vi "HMI.vi"(5 "Disabled?":bool=TRUE, 7 "HMI to Control":T1={"RightDriveValue"=0.0, "LeftDriveValue"=0.0, "Arm Manual "=0.0, "Stacker Manual "=0.0, "Claw Manual "=0.0, "ClawSlightOpenNumber"=0, "Intake Value "=0.0, "Arm States"=enum."4 Tote", "Claw States"=enum."Claw Manual ", "Intake Man. or Sense"=enum."Sensing", "Stacker in Manual?"=FALSE, "Drop Stack? "=FALSE, "Tusk Up Request"=FALSE, "Tusk Down Request"=FALSE, "Inver. Wheels  In Request"=FALSE, "Inverse. Wheels Out Request "=FALSE, "Get Out of Manual Control"=FALSE, "Exit Score State"=FALSE, "DriveStraight Help?"=FALSE, "Stacker Shut Off No."=0, "Stacker Need Off?"=FALSE, "Collecting?"=FALSE, "Go to Hover"=FALSE, "Stack Clamp Lock "=FALSE, "Stack Clamp Unlock "=FALSE, "Claw Intake Value "=0.0, "Stack Clamp Lock No. "=0, "Steal Can (ruin their day?)"=FALSE, "Retract (have mercy?)"=FALSE, "Can Grab No. "=0, "Wench Value to Control "=0.0}, 9 "GamepadData":T5) -> (1 "HMI to Control Out":T1={"RightDriveValue"=0.0, "LeftDriveValue"=0.0, "Arm Manual "=0.0, "Stacker Manual "=0.0, "Claw Manual "=0.0, "ClawSlightOpenNumber"=0, "Intake Value "=0.0, "Arm States"=enum."4 Tote", "Claw States"=enum."Claw Manual ", "Intake Man. or Sense"=enum."Sensing", "Stacker in Manual?"=FALSE, "Drop Stack? "=FALSE, "Tusk Up Request"=FALSE, "Tusk Down Request"=FALSE, "Inver. Wheels  In Request"=FALSE, "Inverse. Wheels Out Request "=FALSE, "Get Out of Manual Control"=FALSE, "Exit Score State"=FALSE, "DriveStraight Help?"=FALSE, "Stacker Shut Off No."=0, "Stacker Need Off?"=FALSE, "Collecting?"=FALSE, "Go to Hover"=FALSE, "Stack Clamp Lock "=FALSE, "Stack Clamp Unlock "=FALSE, "Claw Intake Value "=0.0, "Stack Clamp Lock No. "=0, "Steal Can (ruin their day?)"=FALSE, "Retract (have mercy?)"=FALSE, "Can Grab No. "=0, "Wench Value to Control "=0.0}, 3 "GamepadDataOut":T5)   [LabVIEW 2015]
uses:
  Typedefs/GamepadData.ctl
  Typedefs/HMI_to_Control.ctl
  Typedefs/Arm States.ctl
  Typedefs/ClawStates.ctl
  Typedefs/IntakeWheelSenseOrManual.ctl
  Auton/scriptlib/auto_data.vi
panel:
  in  "Wheel Ramp Step":dbl=1.0 format="%#_13g"
  in  "Throttle Ramp Step":dbl=0.015
  in  "Claw Man Threshold":dbl=0.2
  in  "Throttle Drive Straight Assist Threshold":dbl=0.2
  in  "Wheel Drive Straight Assist Threshold":dbl=0.15
  in  "Man Threshold":dbl=0.3
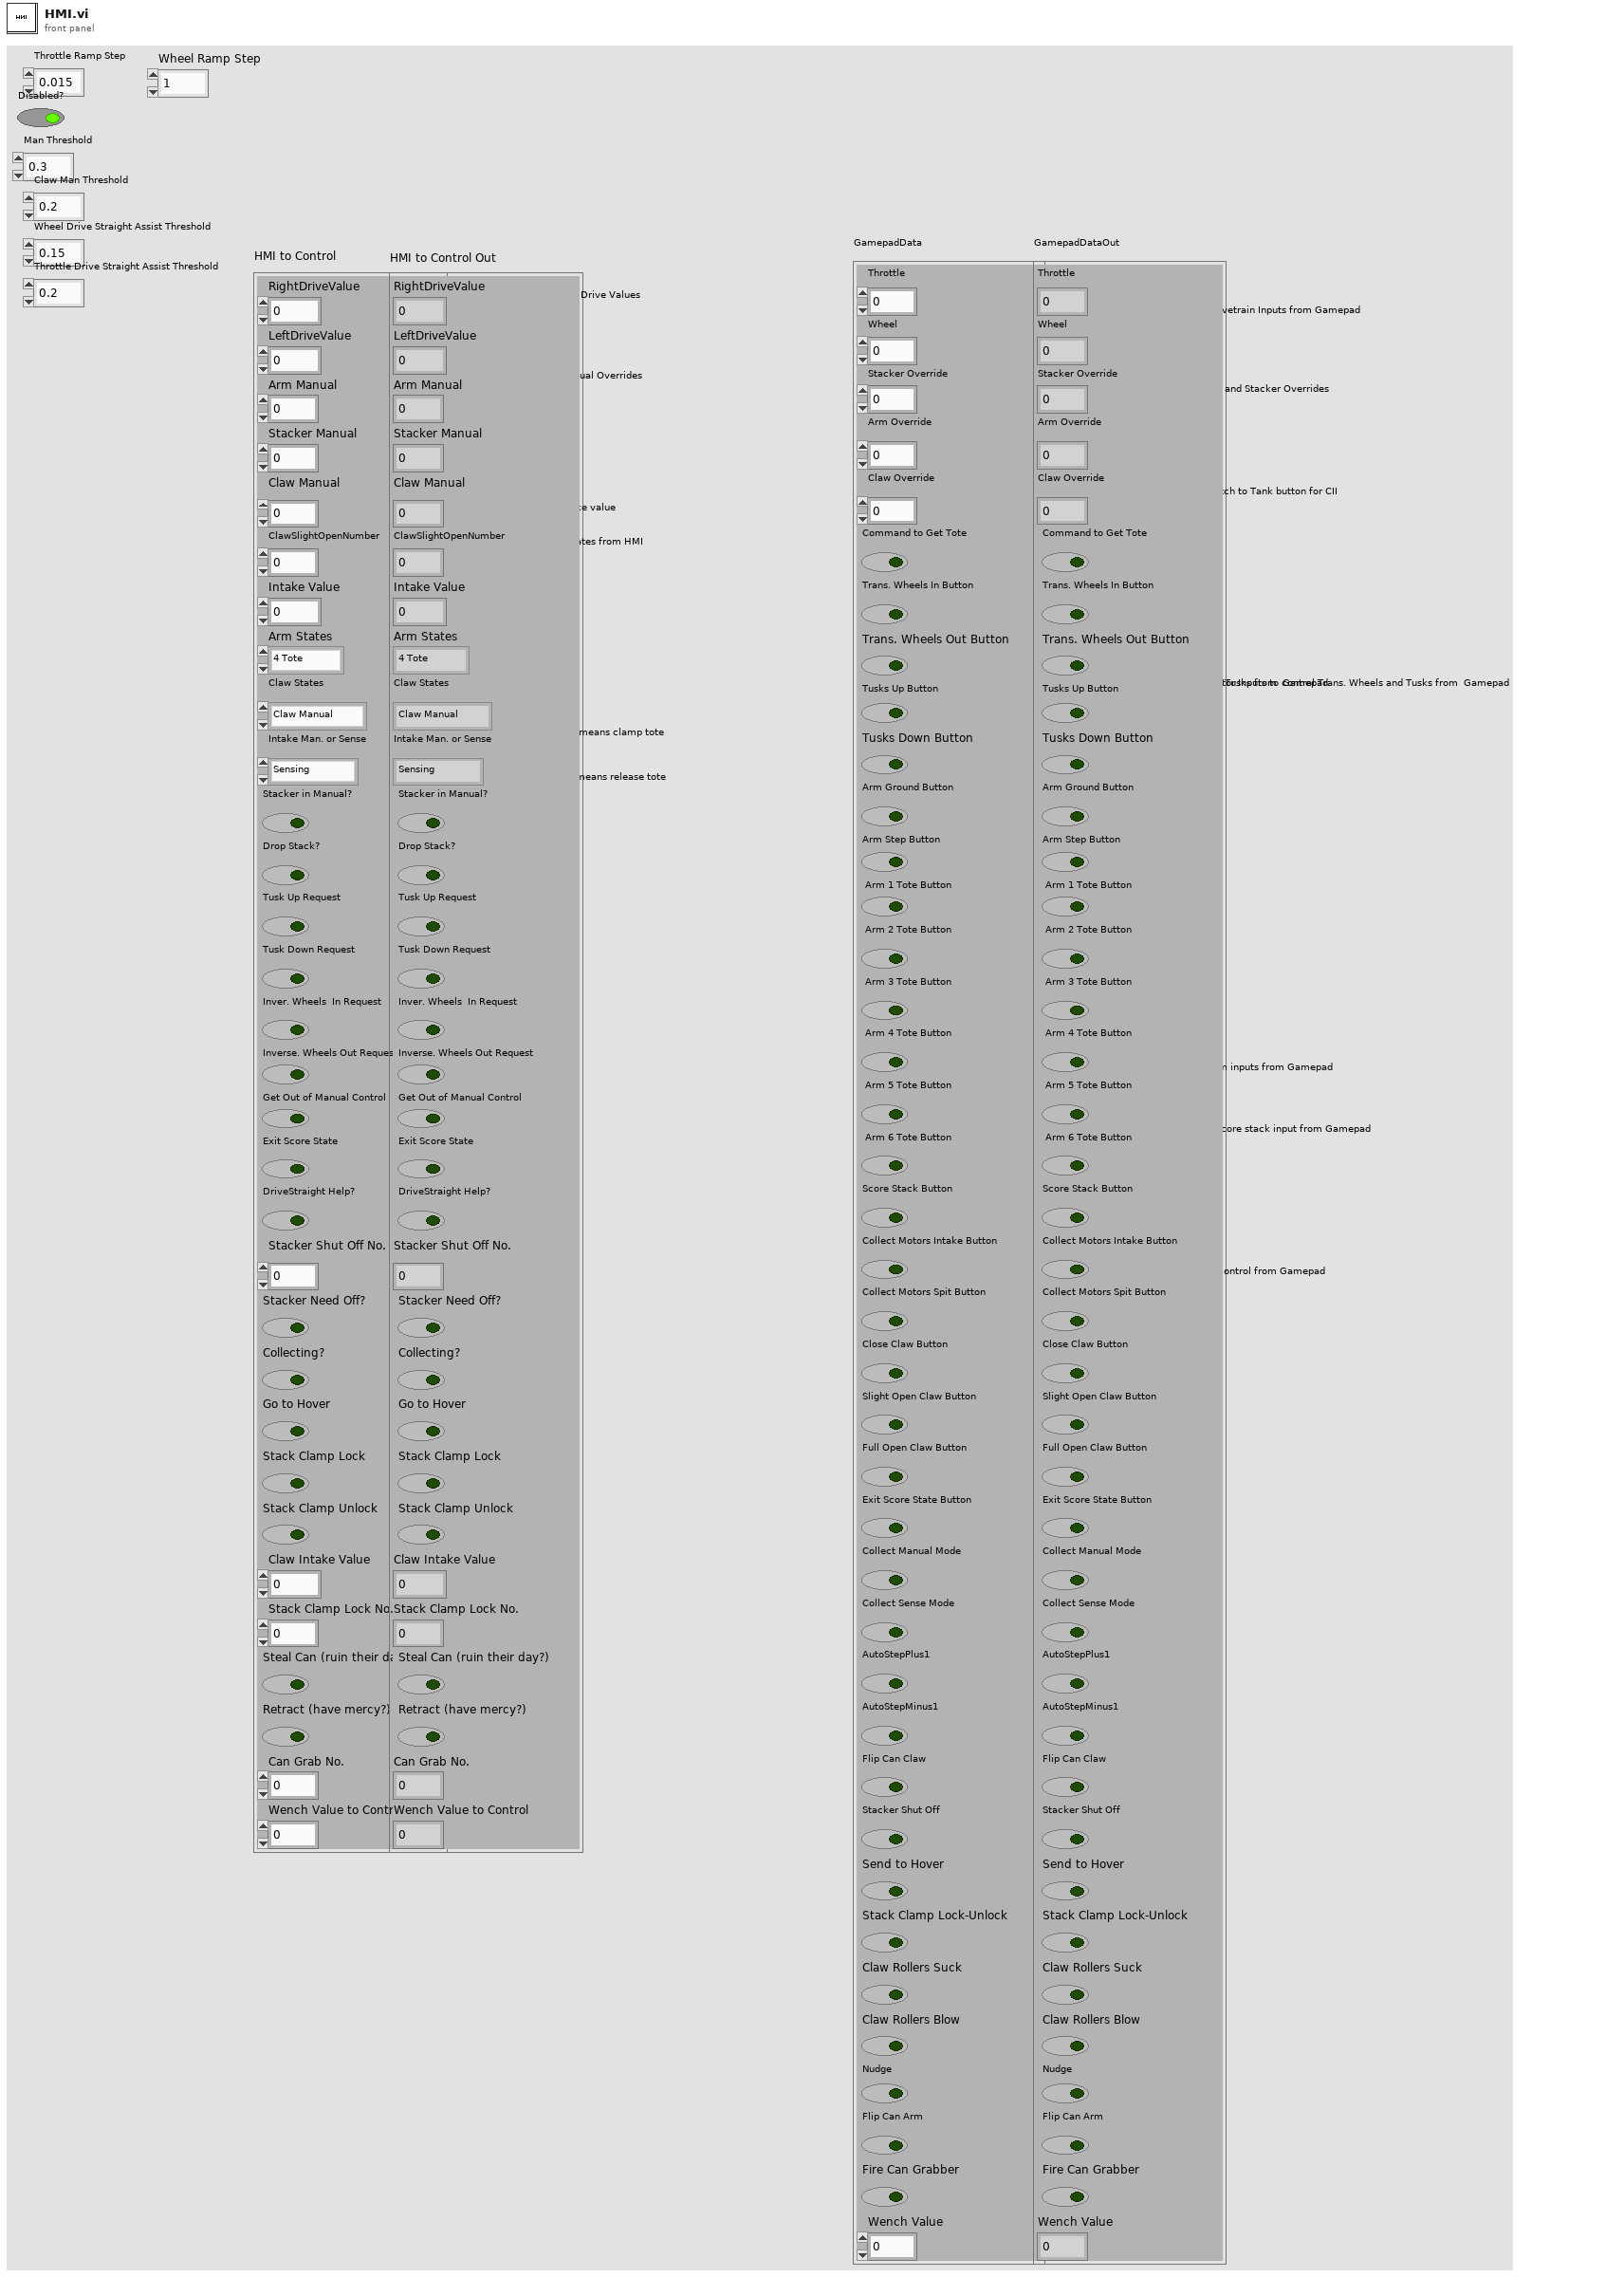
[diagram p1: front panel]
types:
  T1 = typedef "HMI_to_Control.ctl" = cluster{"RightDriveValue":dbl, "LeftDriveValue":dbl, "Arm Manual ":dbl, "Stacker Manual ":dbl, "Claw Manual ":dbl, "ClawSlightOpenNumber":i8, "Intake Value ":sgl, "Arm States":T2, "Claw States":T3, "Intake Man. or Sense":T4, "Stacker in Manual?":bool, "Drop Stack? ":bool, "Tusk Up Request":bool, "Tusk Down Request":bool, "Inver. Wheels  In Request":bool, "Inverse. Wheels Out Request ":bool, "Get Out of Manual Control":bool, "Exit Score State":bool, "DriveStraight Help?":bool, "Stacker Shut Off No.":i8, "Stacker Need Off?":bool, "Collecting?":bool, "Go to Hover":bool, "Stack Clamp Lock ":bool, "Stack Clamp Unlock ":bool, "Claw Intake Value ":sgl, "Stack Clamp Lock No. ":i8, "Steal Can (ruin their day?)":bool, "Retract (have mercy?)":bool, "Can Grab No. ":i8, "Wench Value to Control ":dbl}
  T2 = typedef "Arm States.ctl" = enum16{"Arm Manual ", "Ground", "Step", "1 Tote", "2 Tote", "3 Tote", "4 Tote", "5 Tote", "6 Tote", "Flip Can Arm", "Grab Can in auto", "Nudge"}
  T3 = typedef "ClawStates.ctl" = enum16{"Claw Manual ", "Claw Open", "Claw Closed", "Claw Slight Open", "Flip Can"}
  T4 = typedef "IntakeWheelSenseOrManual.ctl" = enum16{"Sensing", "Manual "}
  T5 = typedef "GamepadData.ctl" = cluster{"Throttle":dbl, "Wheel":dbl, "Stacker Override":dbl, "Arm Override ":dbl, "Claw Override":dbl, "Command to Get Tote":bool, "Trans. Wheels In Button":bool, "Trans. Wheels Out Button":bool, "Tusks Up Button":bool, "Tusks Down Button":bool, "Arm Ground Button":bool, "Arm Step Button":bool, " Arm 1 Tote Button":bool, " Arm 2 Tote Button":bool, " Arm 3 Tote Button ":bool, " Arm 4 Tote Button":bool, " Arm 5 Tote Button":bool, " Arm 6 Tote Button":bool, "Score Stack Button":bool, "Collect Motors Intake Button":bool, "Collect Motors Spit Button":bool, "Close Claw Button":bool, "Slight Open Claw Button":bool, "Full Open Claw Button ":bool, "Exit Score State Button":bool, "Collect Manual Mode ":bool, "Collect Sense Mode":bool, "AutoStepPlus1":bool, "AutoStepMinus1":bool, "Flip Can Claw":bool, "Stacker Shut Off":bool, "Send to Hover ":bool, "Stack Clamp Lock-Unlock ":bool, "Claw Rollers Suck ":bool, "Claw Rollers Blow ":bool, "Nudge":bool, "Flip Can Arm ":bool, "Fire Can Grabber":bool, "Wench Value":dbl}
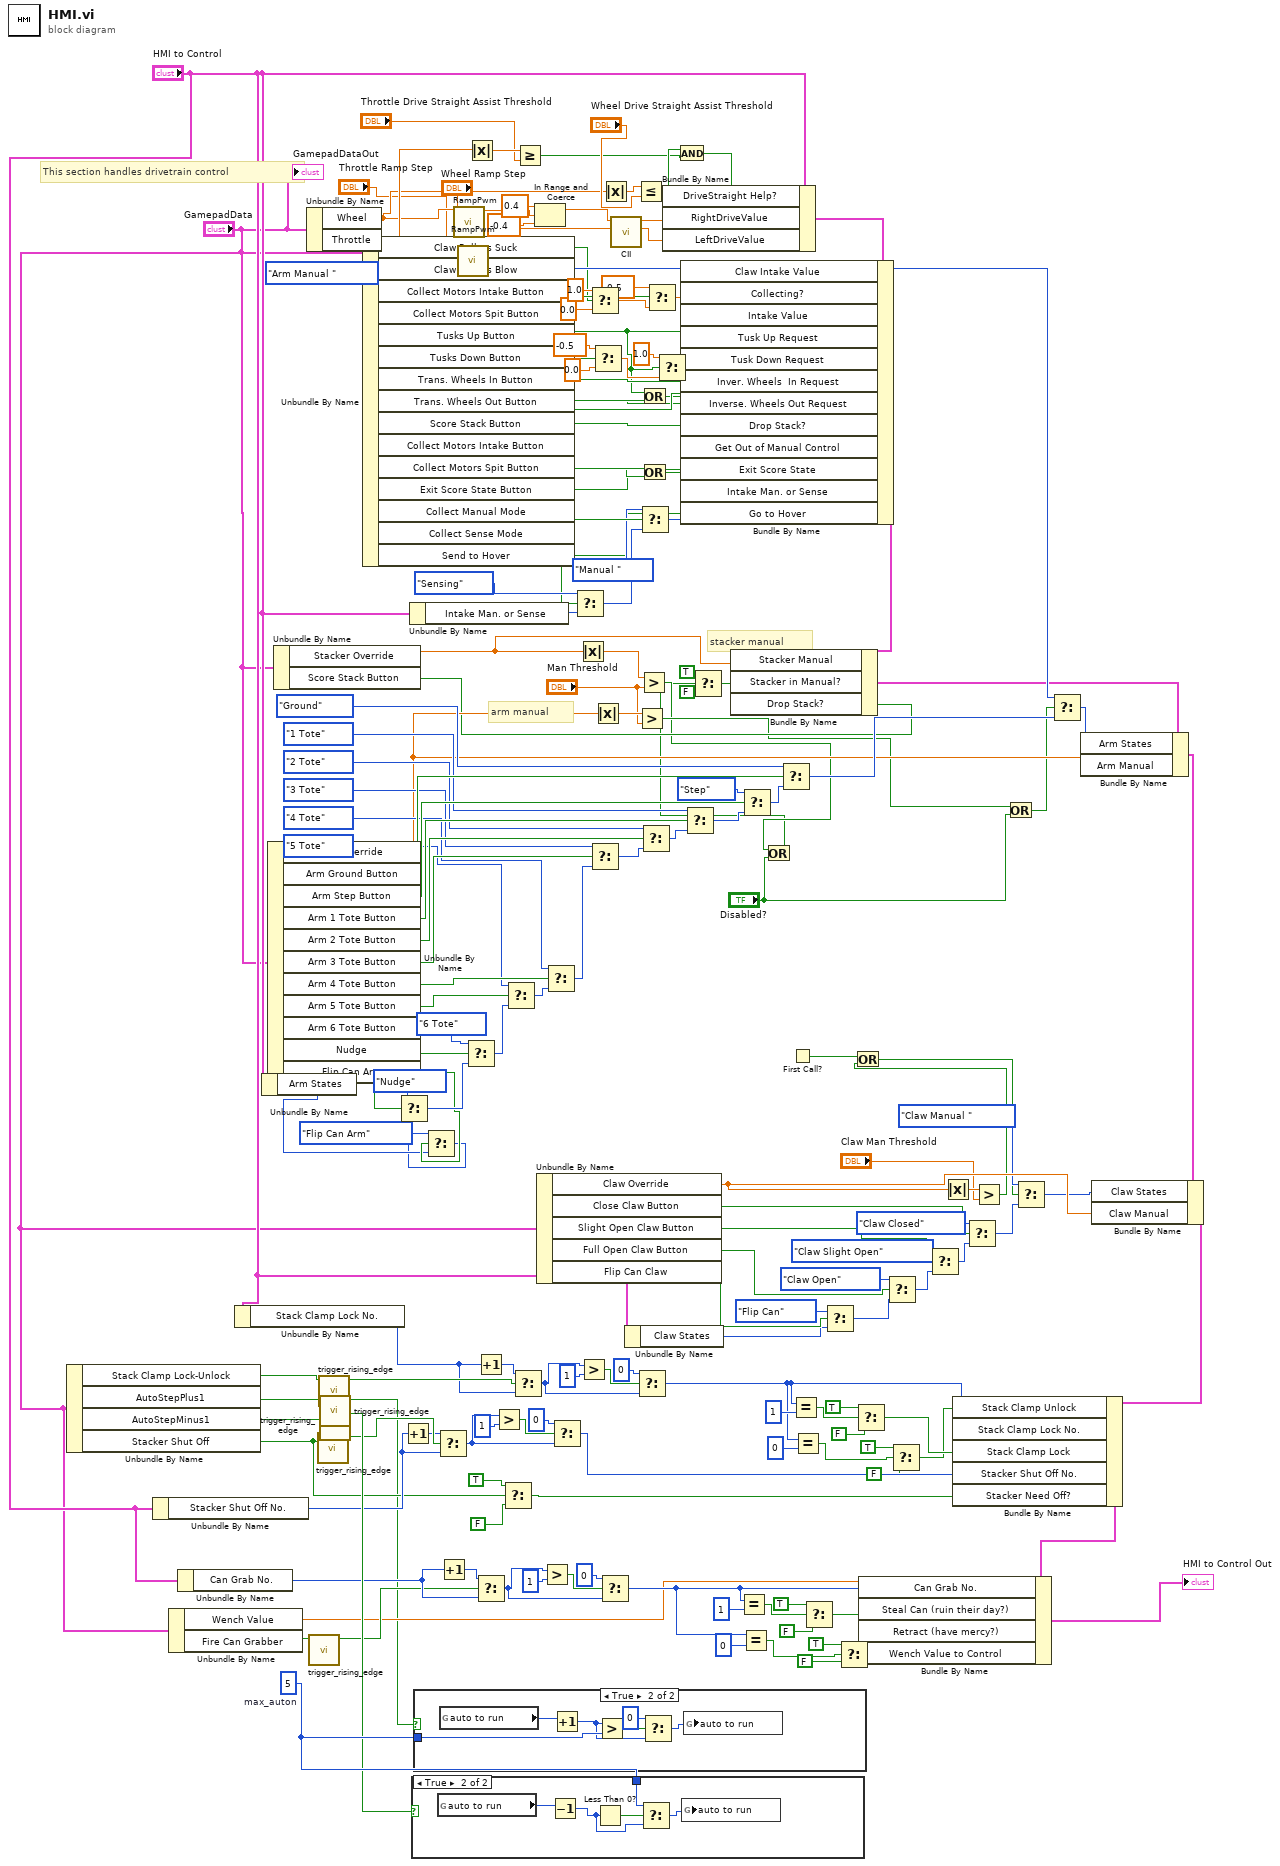
[diagram p0: block diagram]
diagram:
  w91 = i8 5  # max_auton
  # "stacker manual"
  # "arm manual"
  # "This section handles drivetrain control"
  n1 = Unbundle By Name("GamepadData") -> ("Stack Clamp Lock-Unlock"=w60:bool, "AutoStepPlus1"=w93:bool, "AutoStepMinus1"=w92:bool, "Stacker Shut Off"=w76:bool)
  n2 = Unbundle By Name("HMI to Control") -> ("Stacker Shut Off No."=w86:i8)
  n3 = Unbundle By Name("GamepadData") -> ("Wench Value"=w2:dbl, "Fire Can Grabber"=w17:bool)
  n4 = Unbundle By Name("HMI to Control") -> ("Can Grab No."=w19:i8)
  n5 = Unbundle By Name("HMI to Control") -> ("Stack Clamp Lock No."=w57:i8)
  n6 = Unbundle By Name("HMI to Control") -> ("Arm States"=w31:T2)
  n7 = Unbundle By Name("GamepadData") -> ("Arm Override"=w148:dbl, "Arm Ground Button"=w174:bool, "Arm Step Button"=w172:bool, "Arm 1 Tote Button"=w170:bool, "Arm 2 Tote Button"=w167:bool, "Arm 3 Tote Button"=w164:bool, "Arm 4 Tote Button"=w161:bool, "Arm 5 Tote Button"=w158:bool, "Arm 6 Tote Button"=w155:bool, "Nudge"=w34:bool, "Flip Can Arm"=w32:bool)
  n8 = Unbundle By Name("GamepadData") -> ("Stacker Override"=w137:dbl, "Score Stack Button"=w147:bool)
  n9 = Unbundle By Name("GamepadData") -> ("Wheel"=w96:dbl, "Throttle"=w98:dbl)
  n10 = call "trigger_rising_edge.vi"("input"=w17) -> ("rising"=w16:bool)  [unwired: 10 in]
  n11 = call "trigger_rising_edge.vi"("input"=w76) -> ("rising"=w88:bool)  [unwired: 10 in]
  n12 = call "trigger_rising_edge.vi"("input"=w60) -> ("rising"=w58:bool)  [unwired: 10 in]
  n13 = call "trigger_rising_edge.vi"("input"=w93) -> ("rising"=w1:bool)  [unwired: 10 in]
  n14 = call "trigger_rising_edge.vi"("input"=w92) -> ("rising"=w90:bool)  [unwired: 10 in]
  n15 = Unbundle By Name("GamepadData") -> ("Claw Rollers Suck"=w28:bool, "Claw Rollers Blow"=w29:bool, "Collect Motors Intake Button"=w68:bool, "Collect Motors Spit Button"=w176:bool, "Tusks Up Button"=w132:bool, "Tusks Down Button"=w131:bool, "Trans. Wheels In Button"=w122:bool, "Trans. Wheels Out Button"=w121:bool, "Score Stack Button"=w139:bool, "Collect Motors Intake Button"=w136:bool, "Collect Motors Spit Button"=w135:bool, "Exit Score State Button"=w133:bool, "Collect Manual Mode"=w128:bool, "Collect Sense Mode"=w120:bool, "Send to Hover"=w67:bool)
  n16 = Increment(x=w86) -> (x+1=w87:i8)
  n17 = Unbundle By Name("HMI to Control") -> ("Intake Man. or Sense"=w124:T4)
  n18 = case shown="True" w90 {
    tunnel: w91 -> [_ w185]
    frame False {
    }
    frame True {
      n19 = global read "auto_data.vi" "auto to run"() -> (w188:i8)
      n20 = Decrement(x=w188) -> (x-1=w184:i8)
      n21 = Less Than 0?(x=w184) -> (x < 0?=w187:bool)
      n22 = Select(t=w185, s=w187, f=w184) -> (s? t:f=w186:i8)
      n23 = global write "auto_data.vi" "auto to run"(w186) -> ()
    }
  }
  n24 = case shown="True" w1 {
    tunnel: w91 -> [_ w192]
    frame False {
    }
    frame True {
      n25 = global read "auto_data.vi" "auto to run"() -> (w194:i8)
      n26 = Increment(x=w194) -> (x+1=w191:i8)
      n27 = Greater?(x=w191, y=w192) -> (0:w193:bool)
      n28 = Select(t=i8 0, s=w193, f=w191) -> (s? t:f=w189:i8)
      n29 = global write "auto_data.vi" "auto to run"(w189) -> ()
    }
  }
  n30 = Select(t=Arm_States."Flip Can Arm" ("Enum"), s=w32, f=w31) -> (s? t:f=w30:T2)
  n31 = Select(t=Arm_States."Nudge", s=w34, f=w30) -> (s? t:f=w36:T2)
  n32 = Select(t=w87, s=w88, f=w86) -> (s? t:f=w81:i8)
  n33 = Increment(x=w19) -> (x+1=w21:i8)
  n34 = call "RampPwm.vi"("Ramp Step"="Wheel Ramp Step", "Input"=w96) -> ("Output"=w44:dbl)  [unwired: 9 in]
  n35 = call "RampPwm.vi"("Ramp Step"="Throttle Ramp Step", "Input"=w98) -> ("Output"=w97:dbl)  [unwired: 9 in]
  n36 = Select(t=Arm_States."6 Tote" ("Enum"), s=w155, f=w36) -> (s? t:f=w153:T2)
  n37 = Absolute Value(x=w98) -> (abs(x)=w118:dbl)
  n38 = Increment(x=w57) -> (x+1=w59:i8)
  n39 = Select(t=w21, s=w16, f=w19) -> (s? t:f=w20:i8)
  n40 = Greater?(x=w81, y=i8 1) -> (0:w84:bool)
  n41 = Select(t=TRUE, s=w76, f=FALSE) -> (s? t:f=w73:bool)
  n42 = Select(t=Arm_States."5 Tote" ("Enum"), s=w158, f=w153) -> (s? t:f=w156:T2)
  n43 = Select(t=w59, s=w58, f=w57) -> (s? t:f=w56:i8)
  n44 = Greater Or Equal?(x=w118, y="Throttle Drive Straight Assist Threshold") -> (x >= y?=w116:bool)
  n45 = In Range and Coerce(upper limit=0.4, x=w44, lower limit=-0.4) -> (coerced(x)=w41:dbl)  [unwired: 1 out]
  n46 = Unbundle By Name("GamepadData") -> ("Claw Override"=w112:dbl, "Close Claw Button"=w106:bool, "Slight Open Claw Button"=w100:bool, "Full Open Claw Button"=w99:bool, "Flip Can Claw"=w39:bool)
  n47 = Greater?(x=w20, y=i8 1) -> (0:w23:bool)
  n48 = Select(t=Arm_States."4 Tote" ("Enum"), s=w161, f=w156) -> (s? t:f=w160:T2)
  n49 = Select(t=i8 0, s=w84, f=w81) -> (s? t:f=w82:i8)
  n50 = Select(t=IntakeWheelSenseOrManual."Sensing" ("Enum"), s=w120, f=w124) -> (s? t:f=w123:T4)
  n51 = Absolute Value(x=w137) -> (abs(x)=w138:dbl)
  n52 = Greater?(x=w56, y=i8 1) -> (0:w62:bool)
  n53 = Select(t=sgl 1.0, s=w28, f=sgl 0.0) -> (s? t:f=w64:sgl)
  n54 = Select(t=Arm_States."3 Tote" ("Enum"), s=w164, f=w160) -> (s? t:f=w162:T2)
  n55 = Select(t=sgl -0.5, s=w176, f=sgl 0.0) -> (s? t:f=w178:sgl)
  n56 = Absolute Value(x=w148) -> (abs(x)=w152:dbl)
  n57 = Select(t=i8 0, s=w23, f=w20) -> (s? t:f=w5:i8)
  n58 = Absolute Value(x=w96) -> (abs(x)=w129:dbl)
  n59 = call "CII.vi"("Wheel"=w41, "Throttle"=w97) -> ("RightDrive"=w183:dbl, "LeftDrive"=w182:dbl)  [unwired: 7 in]
  n60 = Unbundle By Name("HMI to Control") -> ("Claw States"=w38:T3)
  n61 = Less Or Equal?(x=w129, y="Wheel Drive Straight Assist Threshold") -> (x <= y?=w119:bool)
  n62 = Greater?(x=w152, y="Man Threshold") -> (0:w80:bool)
  n63 = Select(t=i8 0, s=w62, f=w56) -> (s? t:f=w48:i8)
  n64 = Greater?(x=w138, y="Man Threshold") -> (0:w78:bool)
  n65 = Or(x=w68, y=w131) -> (x .or. y?=w130:bool)
  n66 = Or(x=w136, y=w135) -> (x .or. y?=w134:bool)
  n67 = Select(t=IntakeWheelSenseOrManual."Manual " ("Enum"), s=w128, f=w123) -> (s? t:f=w126:T4)
  n68 = Select(t=Arm_States."2 Tote" ("Enum"), s=w167, f=w162) -> (s? t:f=w165:T2)
  n69 = Select(t=sgl -0.5, s=w29, f=w64) -> (s? t:f=w66:sgl)
  n70 = Select(t=sgl 1.0, s=w68, f=w178) -> (s? t:f=w141:sgl)
  n71 = And(x=w119, y=w116) -> (x .and. y?=w115:bool)
  n72 = Bundle By Name(cluster="HMI to Control", "DriveStraight Help?"=w115, "RightDriveValue"=w183, "LeftDriveValue"=w182) -> (w181:T1)
  n73 = Bundle By Name(cluster=w181, "Claw Intake Value"=w66, "Collecting?"=w68, "Intake Value"=w141, "Tusk Up Request"=w132, "Tusk Down Request"=w130, "Inver. Wheels  In Request"=w122, "Inverse. Wheels Out Request"=w121, "Drop Stack?"=w139, "Get Out of Manual Control"=w134, "Exit Score State"=w133, "Intake Man. or Sense"=w126, "Go to Hover"=w67) -> (w140:T1)
  n74 = Select(t=Arm_States."1 Tote" ("Enum"), s=w170, f=w165) -> (s? t:f=w168:T2)
  n75 = Equal?(x=w5, y=i8 1) -> (x = y?=w12:bool)
  n76 = Equal?(x=w5, y=i8 0) -> (x = y?=w6:bool)
  n77 = Select(t=Arm_States."Step" ("Enum"), s=w172, f=w168) -> (s? t:f=w171:T2)
  n78 = Or(x=w78, y="Disabled?") -> (x .or. y?=w77:bool)
  n79 = Select(t=TRUE ("Score Stack Button"), s=w77, f=FALSE ("Score Stack Button")) -> (s? t:f=w143:bool)
  n80 = Bundle By Name(cluster=w140, "Stacker Manual"=w137, "Stacker in Manual?"=w143, "Drop Stack?"=w147) -> (w142:T1)
  n81 = Select(t=Arm_States."Ground" ("Enum"), s=w174, f=w171) -> (s? t:f=w150:T2)
  n82 = First Call?() -> (First Call?: T/F=w69:bool)
  n83 = Equal?(x=w48, y=i8 1) -> (x = y?=w54:bool)
  n84 = Equal?(x=w48, y=i8 0) -> (x = y?=w46:bool)
  n85 = Select(t=TRUE, s=w12, f=FALSE) -> (s? t:f=w4:bool)
  n86 = Select(t=ClawStates."Flip Can" ("Claw States"), s=w39, f=w38) -> (s? t:f=w37:T3)
  n87 = Select(t=TRUE, s=w6, f=FALSE) -> (s? t:f=w3:bool)
  n88 = Select(t=TRUE, s=w54, f=FALSE) -> (s? t:f=w51:bool)
  n89 = Select(t=ClawStates."Claw Open" ("Claw States"), s=w99, f=w37) -> (s? t:f=w103:T3)
  n90 = Select(t=TRUE, s=w46, f=FALSE) -> (s? t:f=w45:bool)
  n91 = Select(t=ClawStates."Claw Slight Open" ("Claw States"), s=w100, f=w103) -> (s? t:f=w102:T3)
  n92 = Absolute Value(x=w112) -> (abs(x)=w111:dbl)
  n93 = Select(t=ClawStates."Claw Closed" ("Claw States"), s=w106, f=w102) -> (s? t:f=w107:T3)
  n94 = Greater?(x=w111, y="Claw Man Threshold") -> (0:w71:bool)
  n95 = Or(x=w69, y=w71) -> (x .or. y?=w70:bool)
  n96 = Or(x=w80, y="Disabled?") -> (x .or. y?=w79:bool)
  n97 = Select(t=ClawStates."Claw Manual " ("Claw States"), s=w70, f=w107) -> (s? t:f=w101:T3)
  n98 = Select(t=Arm_States."Arm Manual " ("Enum"), s=w79, f=w150) -> (s? t:f=w149:T2)
  n99 = Bundle By Name(cluster=w142, "Arm States"=w149, "Arm Manual"=w148) -> (w113:T1)
  n100 = Bundle By Name(cluster=w113, "Claw States"=w101, "Claw Manual"=w112) -> (w89:T1)
  n101 = Bundle By Name(cluster=w89, "Stack Clamp Unlock"=w45, "Stack Clamp Lock No."=w48, "Stack Clamp Lock"=w51, "Stacker Shut Off No."=w82, "Stacker Need Off?"=w73) -> (w15:T1)
  n102 = Bundle By Name(cluster=w15, "Can Grab No."=w5, "Steal Can (ruin their day?)"=w4, "Retract (have mercy?)"=w3, "Wench Value to Control"=w2) -> (→"HMI to Control Out":T1)
  "GamepadDataOut" <- "GamepadData"
